vi "Reset Device Core.vi"(8 "error in (no error)":errorcluster, 11 "CS++Nanotec in":refnum<class "CS++Nanotec.lvclass">) -> (0 "error out":errorcluster, 3 "CS++Nanotec out":refnum<class "CS++Nanotec.lvclass">)   [LabVIEW 2015, in "CS++Nanotec.lvlib" / "CS++Nanotec.lvclass"]
doc: "Perform reset of device."
uses:
  CS++Nanotec.lvclass
  CS++Nanotec.lvclass/CS++Nanotec.ctl
  CSPP_DeviceBase/CS++Motor/CS++Motor.lvclass
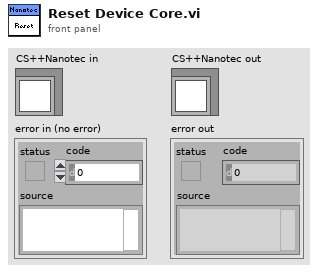
[diagram p1: front panel]
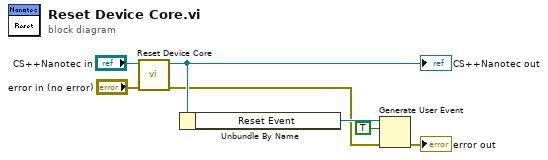
[diagram p0: block diagram]
diagram:
  n1 = call-parent "Reset Device Core.vi"("error in (no error)"="error in (no error)", "CS++Motor in"="CS++Nanotec in") -> ("error out"=w2:errorcluster, "CS++Motor out"=w3:refnum<class "CS++Nanotec.lvclass">)  [unwired: 8 in]
  "CS++Nanotec out" <- w3
  n2 = Unbundle By Name(w3) -> ("Reset Event"=w5:refnum<user-event>)
  n3 = Generate User Event(user event=w5, event data cluster=TRUE ("event data"), error in=w2) -> (error out=→"error out":errorcluster)  [unwired: 1 in, 1 out]
